vi "Get HDD Serial Number.vi"(8 "error in (no error)":errorcluster) -> (0 "error out":errorcluster, 1 "found?":bool, 2 "all serial numbers":string[](array[string]), 3 "disk drive 0 serial number":string)   [LabVIEW 2013]
uses:
  <vilib>/Utility/error.llb/Error Cluster From Error Code.vi
  <vilib>/ErrorRing/Error Ring.xnode
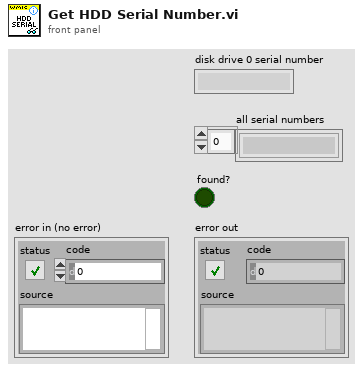
[diagram p1: front panel]
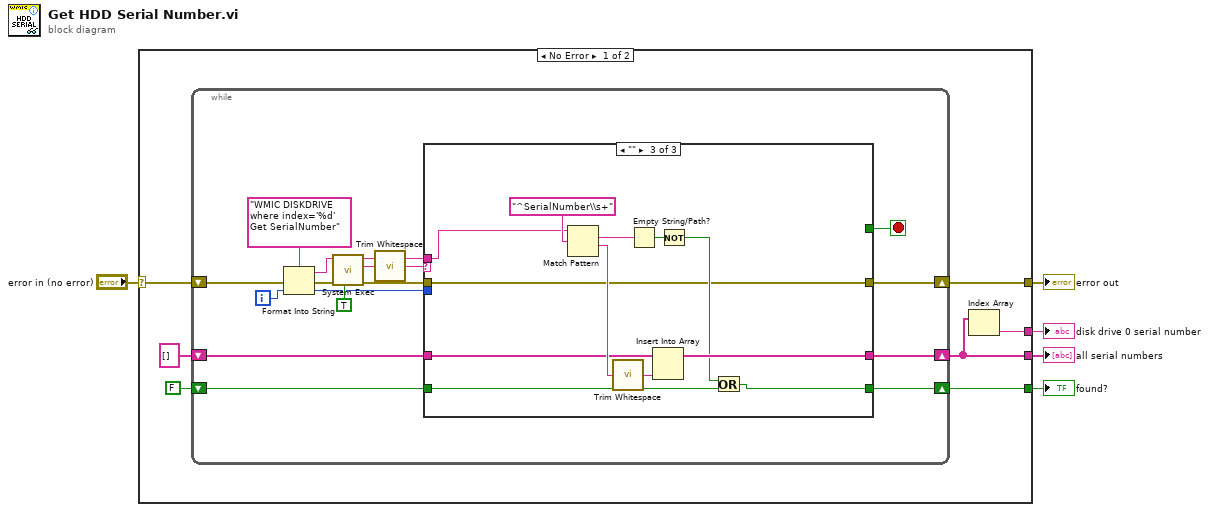
[diagram p0: block diagram]
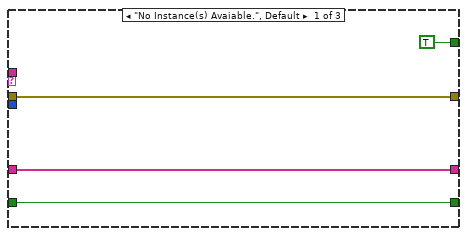
[diagram p2: hidden frame]
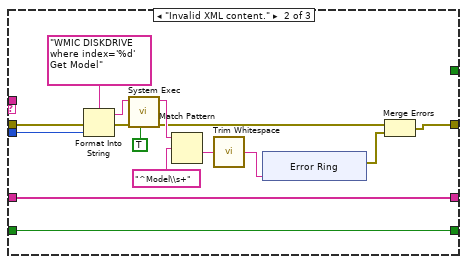
[diagram p3: hidden frame]
diagram:
  n1 = case shown="No Error" "error in (no error)" {
    selector: "error in (no error)" -> [w6 w67]
    tunnel: [w12 _] -> w5
    tunnel: [w11 _] -> w4
    tunnel: [w10 _] -> w3
    tunnel: [w9 w67] -> w2
    frame No Error {
      n2 = while {
        shift-right: [w22] -> w11
        shift-left: string[] [] -> [w21]
        shift-right: [w20] -> w12
        shift-left: FALSE -> [w19]
        shift-right: [w16] -> w9
        shift-left: w6 -> [w15]
        i -> [w17]
        stop <- w13 stop-if-true
        n3 = Format Into String(format string="WMIC DISKDRIVE where index='%d' Get SerialNumber" ("command line"), error in=w15, w17) -> (resulting string=w27:string, error out=w26:errorcluster)  [unwired: 1 in]
        n4 = call <vilib>:"System Exec.vi"("run minimized? (F)"=TRUE, "error in (no error)"=w26, "command line"=w27) -> ("error out"=w18:errorcluster, "standard error"=w25:string, "standard output"=w23:string)  [unwired: 5 in, 1 out]
        n5 = call <vilib>:"Trim Whitespace.vi"("string"=w25) -> ("trimmed string"=w24:string)  [unwired: 1 in]
        n6 = case shown="\"\"" w24 {
          tunnel: w23 -> [_ _ w65]
          tunnel: [w32 w47 w62] -> w22
          tunnel: w21 -> [w32 w47 w61]
          tunnel: [w31 w46 w57] -> w20
          tunnel: w19 -> [w31 w46 w56]
          tunnel: w18 -> [w30 w45 w55]
          tunnel: w17 -> [_ w44 _]
          tunnel: [w30 w34 w55] -> w16
          tunnel: [TRUE _ _] -> w13
          frame "No Instance(s) Avaiable.", Default {
          }
          frame "Invalid XML content." {
            n7 = Format Into String(format string="WMIC DISKDRIVE where index='%d' Get Model" ("command line"), error in=w45, w44) -> (resulting string=w41:string, error out=w42:errorcluster)  [unwired: 1 in]
            n8 = call <vilib>:"System Exec.vi"("run minimized? (F)"=TRUE, "error in (no error)"=w42, "command line"=w41) -> ("error out"=w36:errorcluster, "standard output"=w39:string)  [unwired: 5 in, 2 out]
            n9 = Match Pattern(string=w39, regular expression="^Model\\s+") -> (after substring=w38:string)  [unwired: 1 in, 3 out]
            n10 = call <vilib>:"Trim Whitespace.vi"("string"=w38) -> ("trimmed string"=w37:string)  [unwired: 1 in]
            n11 = xnode "Error Ring"("parameter 0"=w37) -> ("error out"=w35:errorcluster)
            n12 = Merge Errors(w36, w35) -> (w34:errorcluster)
          }
          frame "" {
            n13 = Match Pattern(string=w65, regular expression="^SerialNumber\\s+") -> (match substring=w60:string, after substring=w64:string)  [unwired: 1 in, 2 out]
            n14 = call <vilib>:"Trim Whitespace.vi"("string"=w64) -> ("trimmed string"=w63:string)  [unwired: 1 in]
            n15 = Empty String/Path?(string/path=w60) -> (empty?=w59:bool)
            n16 = Insert Into Array(array=w61, new element=w63) -> (w62:string[])  [unwired: 1 in]
            n17 = Not(x=w59) -> (.not. x?=w58:bool)
            n18 = Or(x=w58, y=w56) -> (x .or. y?=w57:bool)
          }
        }
      }
      n19 = Index Array(array=w11) -> (element=w10:string)  [unwired: 1 in]
    }
    frame Error {
    }
  }
  "found?" <- w5
  "disk drive 0 serial number" <- w3
  "all serial numbers" <- w4
  "error out" <- w2
